vi "Close MeasurementLink Session.vi"(8 "error in":errorcluster, 9 "close session behavior":T1, 10 "session in":variant, 11 "instrument in":refnum<class "Instrument.lvclass">) -> (0 "error out":errorcluster)   [LabVIEW 2020, in "MeasurementLink 34401.lvlib" / "Instrument.lvclass"]
uses:
  Instrument.lvclass
  Instrument.lvclass/Instrument.ctl
  <vilib>/MeasurementLink/MeasurementLink Measurement Server/Helpers/Error Strings Global Internal.vi
  <instrlib>/Agilent 34401/Agilent 34401.lvlib
  <vilib>/MeasurementLink/MeasurementLink Instrument/IInstrument/Close Session Behavior.ctl
  <vilib>/MeasurementLink/MeasurementLink Instrument/IInstrument/IInstrument.lvclass
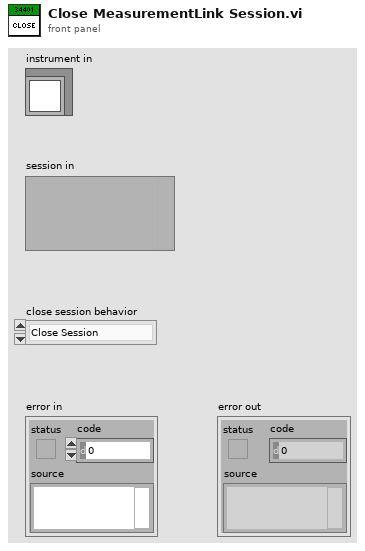
[diagram p1: front panel]
types:
  T1 = typedef "MeasurementLink Instrument.lvlib/IInstrument.lvclass/Close Session Behavior.ctl" = enum16{"Close Session", "Detach Session"}
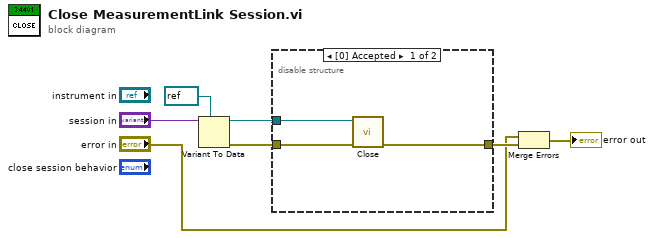
[diagram p0: block diagram]
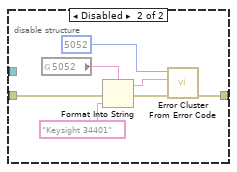
[diagram p2: hidden frame]
diagram:
  n1 = Variant To Data(type=refnum<visa-resource-name> refnum ("VISA resource name out"), Variant="session in") -> (data=w5:refnum<visa-resource-name>, error out=w6:errorcluster)  [unwired: 1 in]
  n2 = disable-structure shown="[0] Accepted" {
    disable-tunnel: w6 -> [w9 w11]
    disable-tunnel: w5 -> [w8 _]
    disable-tunnel: [w10 w17] -> w4
    frame Enabled {
      n3 = call <instrlib>:"Close.vi"("error in (no error)"=w9, "VISA resource name"=w8) -> ("error out"=w10:errorcluster)  [unwired: 9 in]
    }
    frame Disabled {
      n4 = global read "Error Strings Global Internal.vi" "5052"() -> (w15:string)
      n5 = Format Into String(format string=w15, error in=w11, "Keysight 34401") -> (resulting string=w12:string, error out=w13:errorcluster)  [unwired: 1 in]
      n6 = call <vilib>:"Error Cluster From Error Code.vi"("error in (no error)"=w13, "error message (\"\")"=w12, "error code (0)"=5052) -> ("error out"=w17:errorcluster)  [unwired: 6 in]
    }
  }
  n7 = Merge Errors("error in", w4) -> (→"error out":errorcluster)
